vi "Remove Null characters.vi"(2 "String IN":string) -> (16 "String OUT":string)   [LabVIEW 2020, in "Generic Utilities.lvclass"]
uses:
  Generic Utilities.lvclass
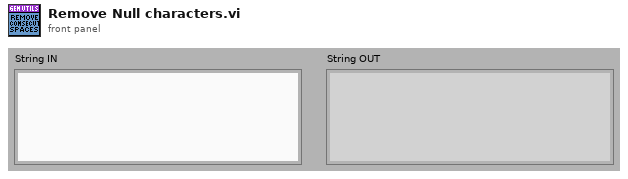
[diagram p1: front panel]
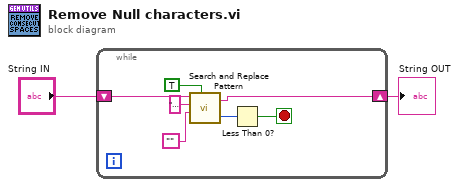
[diagram p0: block diagram]
diagram:
  n1 = while {
    shift-right: [w6] -> w1
    shift-left: "String IN" -> [w9]
    stop <- w4 stop-if-true
    n2 = call <vilib>:"Search and Replace Pattern.vi"("string"=w9, "regular expression (\"\")"="\u0000" ("regular expression (\"\")"), "replace string (\"\")"="", "replace all? (F)"=TRUE) -> ("result string"=w6:string, "offset past match"=w5:i32)  [unwired: 1 in]
    n3 = Less Than 0?(x=w5) -> (x < 0?=w4:bool)
  }
  "String OUT" <- w1
